vi "Get number of pages.vi"(8 "error in (no error)":errorcluster, 11 "TIFF File ref":i32) -> (0 "error out":errorcluster, 2 "Number of Pages":i32, 3 "TIFF File ref out":i32)   [LabVIEW 2012]
uses:
  VisualCPP/LabTIFF/Release/LabTIFF.dll
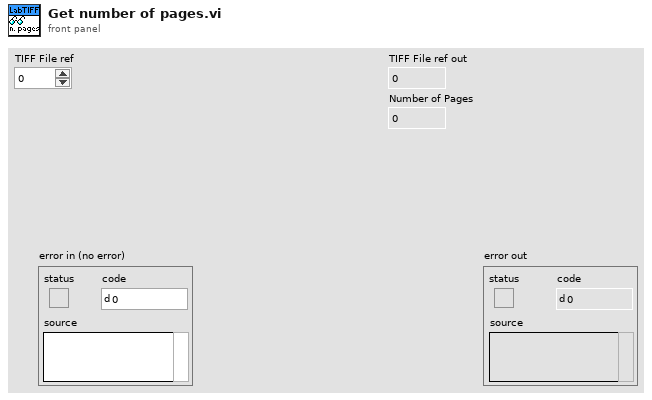
[diagram p1: front panel]
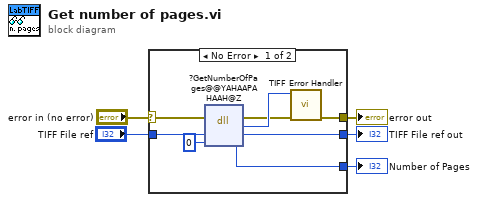
[diagram p0: block diagram]
diagram:
  n1 = case shown="No Error" "error in (no error)" {
    selector: "error in (no error)" -> [w13 w15]
    tunnel: "TIFF File ref" -> [w12 w14]
    tunnel: [w8 w14] -> w3
    tunnel: [w7 _] -> w1
    tunnel: [w6 w15] -> w2
    frame No Error {
      n2 = dll-call lib="C:/Users/Ludovico/Prog/moroder/dependencies/LabTIFF/VisualCPP/LabTIFF/Release/LabTIFF.dll" fn="?GetNumberOfPages@@YAHAAPAHAAH@Z"(error in=w13, "File Reference"=w12, "Number of Pages"=0) -> (error out=w9:errorcluster, "error"=w10:i32, "File Reference"=w8:i32, "Number of Pages"=w7:i32)  [unwired: 2 in, 1 out]
      n3 = call "TIFF Error Handler.vi"("error in (no error)"=w9, "TIFF DLL error"=w10) -> ("error out"=w6:errorcluster)  [unwired: 9 in]
    }
    frame Error {
    }
  }
  "error out" <- w2
  "TIFF File ref out" <- w3
  "Number of Pages" <- w1
